vi "ToVisaResourceName.vi"(8 "error in":errorcluster, 11 "Generic":refnum<class "Generic.lvclass">) -> (0 "error out":errorcluster, 3 "VisaResourceName":refnum<class "VisaResourceName.lvclass">)   [LabVIEW 2014, in "Raspberry Pi Compatible Compiler for LabVIEW.lvlib" / "VisaResourceName.lvclass"]
uses:
  VisaResourceName.lvclass
  Generic/Generic.lvclass
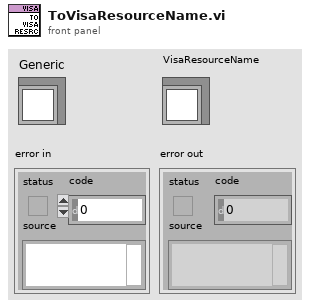
[diagram p1: front panel]
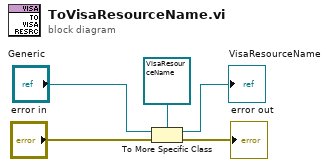
[diagram p0: block diagram]
diagram:
  n1 = To More Specific Class(target class=refnum<class "VisaResourceName.lvclass"> refnum ("Numeric in"), reference="Generic", error in="error in") -> (specific class reference=→"VisaResourceName":refnum<class "VisaResourceName.lvclass">, error out=→"error out":errorcluster)
